vi "StopAndWaitForIdle.vi"(11 "error in (no error)":errorcluster) -> (3 "error out":errorcluster, 5 "Changed?":bool)   [LabVIEW 2018, in "SyncModule.lvlib"]
uses:
  SyncModule.lvlib
  <vilib>/Utility/error.llb/Error Cluster From Error Code.vi
  <vilib>/ErrorRing/Error Ring.xnode
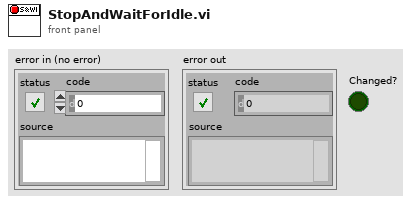
[diagram p1: front panel]
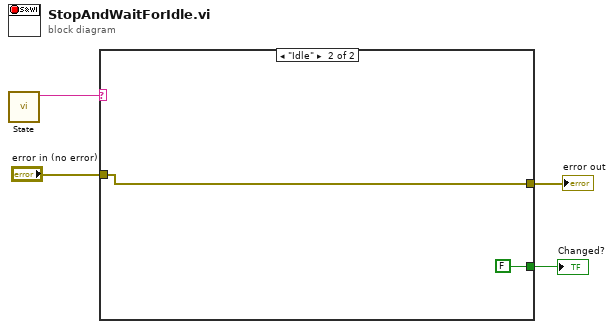
[diagram p0: block diagram]
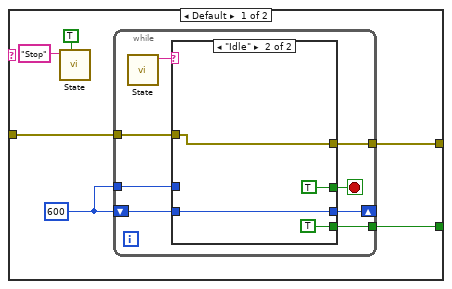
[diagram p2: hidden frame]
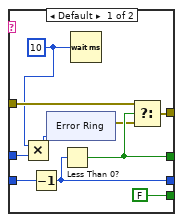
[diagram p3: hidden frame]
diagram:
  n1 = call "State.vi"() -> ("State"=w4:string)  [unwired: 11 in]
  n2 = case shown="\"Idle\"" w4 {
    tunnel: "error in (no error)" -> [w8 w41]
    tunnel: [w6 w41] -> w2
    tunnel: [w5 FALSE] -> w1
    frame Default {
      w7 = 600
      n3 = call "State.vi"("Set (f)"=TRUE, "State"="Stop") -> ()  [unwired: 9 in, 1 out]
      n4 = while {
        tunnel: w8 -> [w17]
        shift-right: [w15] -> _
        shift-left: w7 -> [w16]
        tunnel: w7 -> [w13]
        tunnel: [w12] -> w6
        tunnel: [w11] -> w5
        stop <- w14 stop-if-true
        n5 = call "State.vi"() -> ("State"=w18:string)  [unwired: 11 in]
        n6 = case shown="\"Idle\"" w18 {
          tunnel: w17 -> [w26 w37]
          tunnel: w16 -> [w28 w38]
          tunnel: [w27 w38] -> w15
          tunnel: [w25 TRUE] -> w14
          tunnel: w13 -> [w24 _]
          tunnel: [w20 w37] -> w12
          tunnel: [FALSE TRUE] -> w11
          frame Default {
            w23 = u32 10 ("milliseconds to wait")
            n7 = Multiply(x=w23, y=w24) -> (x*y=w22:u32)
            n8 = Decrement(x=w28) -> (x-1=w27:i32)
            n9 = xnode "Error Ring"("parameter 0"=w22) -> ("error out"=w21:errorcluster)
            n10 = Less Than 0?(x=w27) -> (x < 0?=w25:bool)
            n11 = Wait (ms)(milliseconds to wait=w23) -> ()  [unwired: 1 out]
            n12 = Select(t=w26, s=w25, f=w21) -> (s? t:f=w20:errorcluster)
          }
          frame "Idle" {
          }
        }
      }
    }
    frame "Idle" {
    }
  }
  "error out" <- w2
  "Changed?" <- w1
